vi "xps_panel_DO_move_stage_absolute.vi"(8 "error in (no error)":errorcluster, 10 "Position":dbl, 11 "newport_xps_panel in":refnum<class "newport_xps_panel.lvclass">) -> (0 "error out":errorcluster, 3 "newport_xps_panel out":refnum<class "newport_xps_panel.lvclass">)   [LabVIEW 2015, in "newport_xps_panel.lvclass"]
uses:
  newport_xps_panel.lvclass
  newport_xps/newport_xps.lvclass
  UI/panel_class/panel.lvclass
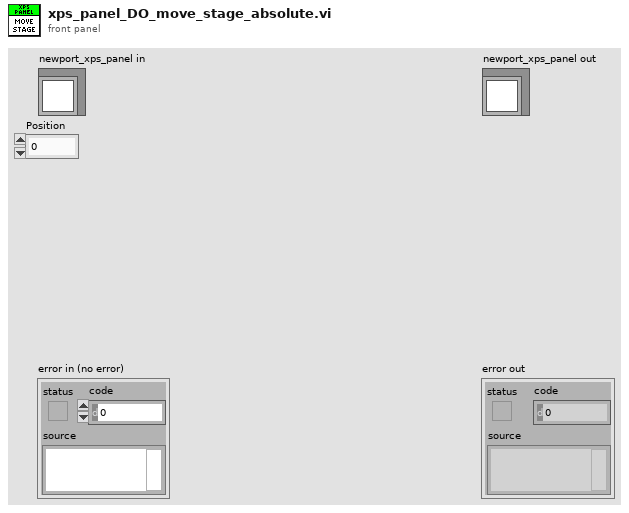
[diagram p1: front panel]
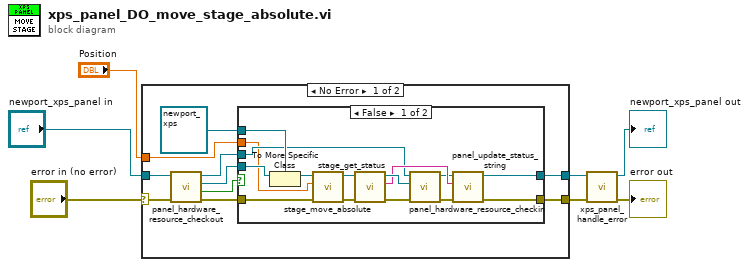
[diagram p0: block diagram]
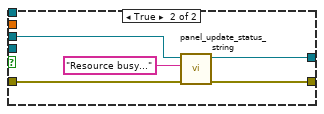
[diagram p2: hidden frame]
diagram:
  n1 = case shown="No Error" "error in (no error)" {
    selector: "error in (no error)" -> [w17 w39]
    tunnel: [w8 w39] -> w4
    tunnel: [w9 w38] -> w3
    tunnel: "newport_xps_panel in" -> [w16 w38]
    tunnel: "Position" -> [w10 _]
    frame No Error {
      n2 = call "panel_hardware_resource_checkout.vi"("error in (no error)"=w17, "panel in"=w16) -> ("error out"=w12:errorcluster, "timed out?"=w15:bool, "hardware.lvclass"=w13:refnum<class "hardware.lvclass">, "panel out"=w14:refnum<class "newport_xps_panel.lvclass">)  [unwired: 6 in]
      n3 = case shown="False" w15 {
        tunnel: w14 -> [w22 w34]
        tunnel: w13 -> [w32 _]
        tunnel: w12 -> [w25 w37]
        tunnel: [w19 w36] -> w8
        tunnel: [w18 w33] -> w9
        tunnel: refnum<class "newport_xps.lvclass"> refnum ("newport_xps in") -> [w31 _]
        tunnel: w10 -> [w20 _]
        frame False {
          n4 = To More Specific Class(target class=w31, reference=w32) -> (specific class reference=w21:refnum<class "newport_xps.lvclass">)  [unwired: 1 in, 1 out]
          n5 = call-dynamic "stage_move_absolute.vi"("error in (no error)"=w25, "Position"=w20, "newport_xps in"=w21) -> ("error out"=w24:errorcluster, "newport_xps out"=w23:refnum<class "newport_xps.lvclass">)  [unwired: 7 in]
          n6 = call-dynamic "stage_get_status.vi"("error in (no error)"=w24, "newport_xps in"=w23) -> ("error out"=w26:errorcluster, "Status"=w28:string, "newport_xps out"=w29:refnum<class "newport_xps.lvclass">)  [unwired: 7 in]
          n7 = call "panel_hardware_resource_checkin.vi"("error in (no error)"=w26, "hardware.lvclass"=w29, "panel in"=w22) -> ("error out"=w30:errorcluster, "panel out"=w27:refnum<class "newport_xps_panel.lvclass">)  [unwired: 7 in]
          n8 = call-dynamic "panel_update_status_string.vi"("error in (no error)"=w30, "String"=w28, "newport_xps_panel in"=w27) -> ("error out"=w19:errorcluster, "newport_xps_panel out"=w18:refnum<class "newport_xps_panel.lvclass">)  [unwired: 7 in]
        }
        frame True {
          n9 = call-dynamic "panel_update_status_string.vi"("error in (no error)"=w37, "String"="Resource busy...", "newport_xps_panel in"=w34) -> ("error out"=w36:errorcluster, "newport_xps_panel out"=w33:refnum<class "newport_xps_panel.lvclass">)  [unwired: 7 in]
        }
      }
    }
    frame Error {
    }
  }
  n10 = call "xps_panel_handle_error.vi"("error in (no error)"=w4, "newport_xps_panel in"=w3) -> ("error out"=→"error out":errorcluster, "newport_xps_panel out"=→"newport_xps_panel out":refnum<class "newport_xps_panel.lvclass">)  [unwired: 8 in]
